vi "QueryBCMOut.vi"(8 "error in (no error)":errorcluster, 10 "Timeout(s)":dbl, 11 "COM Port":refnum<visa-resource-name>="COM3") -> (0 "error out":errorcluster, 2 "BCMOut":i32, 3 "COM Port Out":refnum<visa-resource-name>="COM3")   [LabVIEW 2020]
uses:
  <userlib>/_OpenG.lib/array/array.llb/Empty 1D Array (String)__ogtk.vi
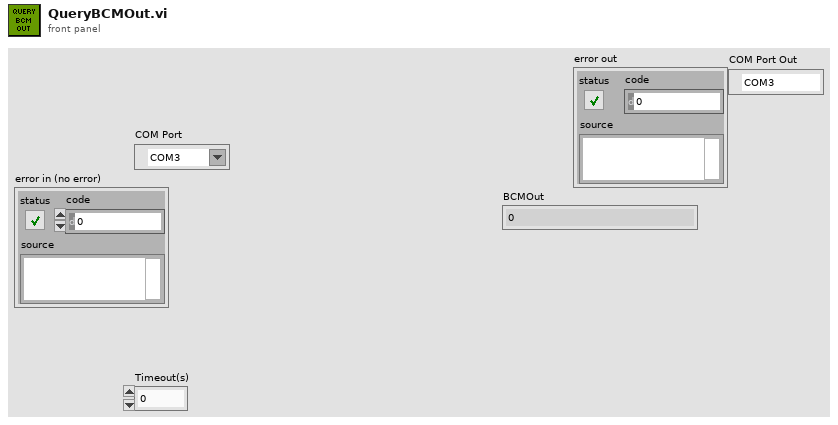
[diagram p1: front panel]
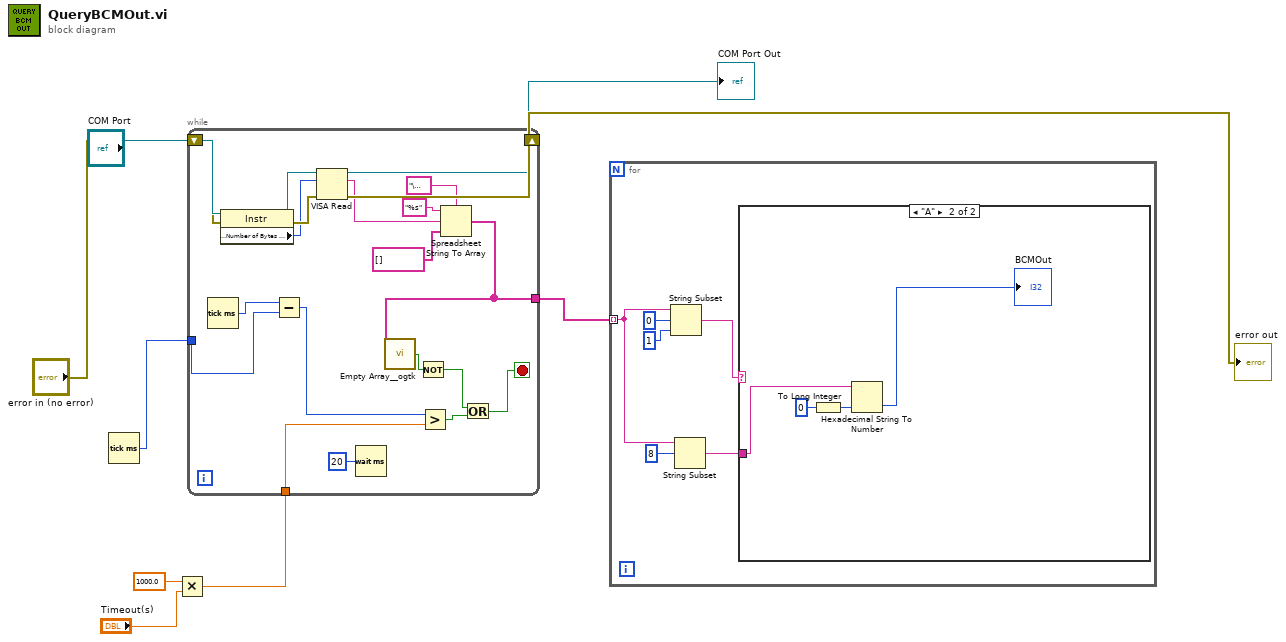
[diagram p0: block diagram]
diagram:
  n1 = Tick Count (ms)() -> (millisecond timer value=w4:u32)
  n2 = Multiply(x=1000.0, y="Timeout(s)") -> (x*y=w1:dbl)
  n3 = while {
    tunnel: [w19] -> w5
    shift-right: [w20] -> w6
    shift-left: "COM Port" -> [w30]
    shift-right: [w28] -> w7
    shift-left: "error in (no error)" -> [w29]
    tunnel: w4 -> [w15]
    tunnel: w1 -> [w13]
    stop <- w10 stop-if-true
    n4 = Tick Count (ms)() -> (millisecond timer value=w16:u32)
    n5 = property class="Instr"(reference=w30, error in=w29) -> (reference out=w23:refnum<visa-resource-name>, error out=w22:errorcluster, "Serial Settings:Number of Bytes at Serial Port"=w21:u32)
    n6 = Subtract(x=w16, y=w15) -> (x-y=w14:u32)
    n7 = VISA Read(VISA resource name=w23, byte count=w21, error in (no error)=w22) -> (VISA resource name out=w20:refnum<visa-resource-name>, read buffer=w26:string, error out=w28:errorcluster)  [unwired: 1 out]
    n8 = Wait (ms)(milliseconds to wait=u32 20) -> ()  [unwired: 1 out]
    n9 = Greater?(x=w14, y=w13) -> (0:w12:bool)
    n10 = Spreadsheet String To Array(delimiter (Tab)="\u0000", format string="%s", spreadsheet string=w26, array type (2D Dbl)=string[] []) -> (array=w19:string[])
    n11 = call-poly <userlib>:"Empty Array__ogtk.vi"("Array"=w19) -> ("Empty Array?"=w18:bool)  [unwired: 8 in]
    n12 = Not(x=w18) -> (.not. x?=w11:bool)
    n13 = Or(x=w11, y=w12) -> (x .or. y?=w10:bool)
  }
  "error out" <- w7
  "COM Port Out" <- w6
  n14 = for {
    tunnel: w5 -> [w33] mode=indexing
    n15 = String Subset(string=w33, offset (0)=0 ("index"), length (rest)=1 ("length")) -> (substring=w32:string)
    n16 = String Subset(string=w33, offset (0)=8 ("index")) -> (substring=w31:string)  [unwired: 1 in]
    n17 = case shown="\"A\"" w32 {
      tunnel: w31 -> [_ w38]
      frame "False", Default {
      }
      frame "A" {
        n18 = To Long Integer(number=0 ("default (0 U32)")) -> (32bit integer=w40:i32)
        n19 = Hexadecimal String To Number(string=w38, default (0uL)=w40) -> (number=→"BCMOut":i32)  [unwired: 1 in, 1 out]
      }
    }
  }
